vi "FestoCPX.Valve(1out1in).vi"(4 "negate input (F)":bool, 6 "Timeout [ms] (5000)":u32=5000, 8 "error in (no error)":errorcluster, 9 "Position":T3, 10 "Output":T1, 11 "Input":T2) -> (0 "error out":errorcluster, 2 "Aborted?":bool, 3 "Timeout?":bool)   [LabVIEW 2016]
uses:
  Station/Station.ValvePosition.ctl
  FestoCPX.DI.Signal.ctl
  FestoCPX.DO.Signal.ctl
  FestoCPX.DO.Data.State.Set.vi
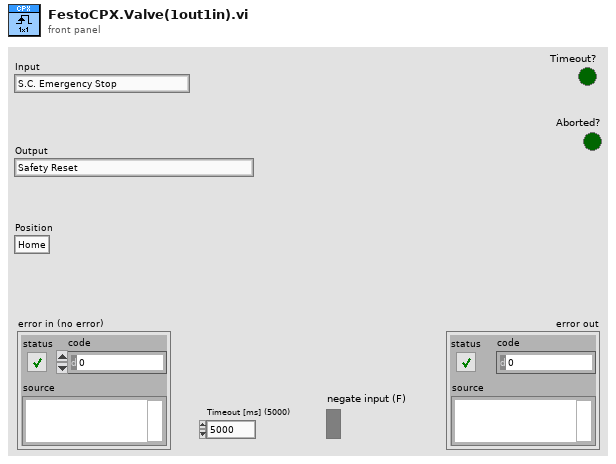
[diagram p1: front panel]
types:
  T1 = typedef "FestoCPX.DO.Signal.ctl" = enum16{"Safety Reset", "Air Main Valve", "Door Lock", "Button LED Start", "Button LED Stop", "Button LED Control", "Traffic LED Red", "Traffic LED Orange", "Traffic LED Green", "Horn", "Laser Interlock", "Laser Trigger", "Laser Fume Extractor", "Product Suction Gripper Slot 1 A", "Product Suction Gripper Slot 1 B", "Product Suction Gripper Slot 2 A", "Product Suction Gripper Slot 2 B", "Product Suction Gripper Slot 3 A", "Product Suction Gripper Slot 3 B", "Product Suction Gripper Slot 4 A", "Product Suction Gripper Slot 4 B", "Product Suction Gripper Final A", "Product Suction Gripper Final B", "Lamp", "Q1 Product Move Work", "Q1 Product Move Home", "Q2 Table Turn Work", "Q2 Table Turn Home", "Q3 Product Lift A", "Q3 Product Lift B", "Q4 Product Arm OK", "Q4 Product Arm NOK", "Q5 Product Arm Work", "Q6 Product BlowOut A", "Q6 Product BlowOut B"}
  T2 = typedef "FestoCPX.DI.Signal.ctl" = enum16{"S.C. Emergency Stop", "S.C. Side Door Close", "S.C. Front Door Close", "S.C. Front Door Secured", "Button Start", "Button Stop", "Button Control", "Product Move Home", "Product Move Work", "Table Position", "Table Lock", "Product Lift A Home", "Product Lift B Home", "Product Arm OK", "Product Arm NOK", "Product Arm Work", "Revolver ID 1", "Revolver ID 2", "Revolver ID 3", "Revolver ID 4", "Revolver ID 5", "Air Pressure Inside", "Air Pressure Inlet", "Product Slot 1 A Present", "Product Slot 1 B Present", "Product Slot 2 A Present", "Product Slot 2 B Present", "Product Slot 3 A Present", "Product Slot 3 B Present", "Product Slot 4 A Present", "Product Slot 4 B Present", "Product Final A Present", "Product Final B Present", "Product Output A Present", "Product Output B Present", "Product Container OK Present", "Product Container NOK Present", "Fork ID 1", "Fork ID 2"}
  T3 = typedef "Station.ValvePosition.ctl" = enum16{"Home", "Work"}
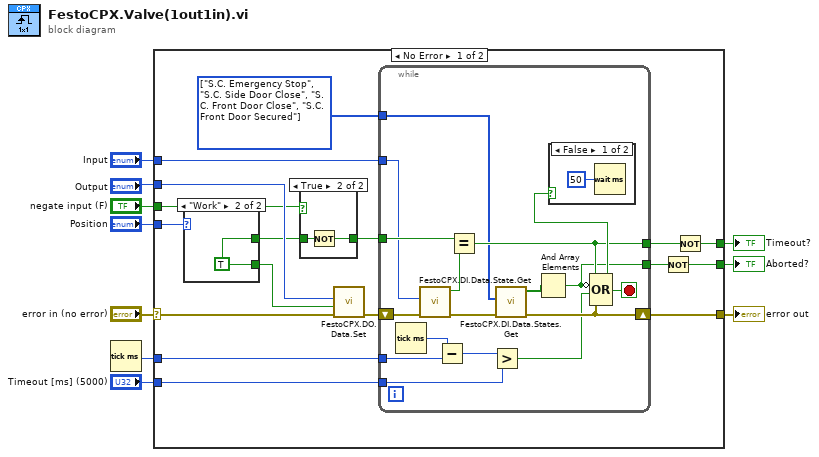
[diagram p0: block diagram]
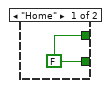
[diagram p3: hidden frame]
diagram:
  n1 = Tick Count (ms)() -> (millisecond timer value=w6:u32)
  n2 = case shown="No Error" "error in (no error)" {
    selector: "error in (no error)" -> [w21 w50]
    tunnel: "Position" -> [w20 _]
    tunnel: [w17 w50] -> w9
    tunnel: [w24 _] -> w8
    tunnel: w6 -> [w27 _]
    tunnel: "Timeout [ms] (5000)" -> [w26 _]
    tunnel: "Input" -> [w25 _]
    tunnel: "Output" -> [w18 _]
    tunnel: [w14 _] -> w2
    tunnel: "negate input (F)" -> [w13 _]
    frame No Error {
      w15 = T2[] [enum."S.C. Emergency Stop", enum."S.C. Side Door Close", enum."S.C. Front Door Close", enum."S.C. Front Door Secured"] items=["S.C. Emergency Stop", "S.C. Side Door Close", "S.C. Front Door Close", "S.C. Front Door Secured", "Button Start", "Button Stop", "Button Control", "Product Move Home", "Product Move Work", "Table Position", "Table Lock", "Product Lift A Home", "Product Lift B Home", "Product Arm OK", "Product Arm NOK", "Product Arm Work", "Revolver ID 1", "Revolver ID 2", "Revolver ID 3", "Revolver ID 4", "Revolver ID 5", "Air Pressure Inside", "Air Pressure Inlet", "Product Slot 1 A Present", "Product Slot 1 B Present", "Product Slot 2 A Present", "Product Slot 2 B Present", "Product Slot 3 A Present", "Product Slot 3 B Present", "Product Slot 4 A Present", "Product Slot 4 B Present", "Product Final A Present", "Product Final B Present", "Product Output A Present", "Product Output B Present", "Product Container OK Present", "Product Container NOK Present", "Fork ID 1", "Fork ID 2"] ("CPX.DI")
      n3 = case shown="\"Work\"" w20 {
        tunnel: [w31 w32] -> w12
        tunnel: [w31 w32] -> w19
        frame "Home" {
          w31 = FALSE
        }
        frame "Work" {
          w32 = TRUE
        }
      }
      n4 = case shown="True" w13 {
        tunnel: w12 -> [w28 w30]
        tunnel: [w28 w29] -> w11
        frame False {
        }
        frame True {
          n5 = Not(x=w30) -> (.not. x?=w29:bool)
        }
      }
      n6 = call-poly "FestoCPX.DO.Data.Set.vi"("error in (no error)"=w21, "State"=w19, "CPX.DO"=w18) -> ("error out"=w23:errorcluster)  [unwired: 8 in]
      n7 = while {
        shift-right: [w37] -> w17
        shift-left: w23 -> [w42]
        tunnel: w25 -> [w40]
        tunnel: [w41] -> w22
        tunnel: w27 -> [w47]
        tunnel: w26 -> [w45]
        tunnel: w11 -> [w44]
        tunnel: [w36] -> w16
        tunnel: w15 -> [w38]
        stop <- w43 stop-if-true
        n8 = Tick Count (ms)() -> (millisecond timer value=w48:u32)
        n9 = call "FestoCPX.DI.Data.State.Get.vi"("error in (no error)"=w42, "CPX.DI"=w40) -> ("error out"=w39:errorcluster, "State"=w33:bool)  [unwired: 5 in, 3 out]
        n10 = Subtract(x=w48, y=w47) -> (x-y=w46:u32)
        n11 = Equal?(x=w44, y=w33) -> (x = y?=w41:bool)
        n12 = Greater?(x=w46, y=w45) -> (0:w35:bool)
        n13 = call "FestoCPX.DI.Data.States.Get.vi"("error in (no error)"=w39, "CPX.DI"=w38) -> ("error out"=w37:errorcluster, "State"=w34:bool[])  [unwired: 5 in, 3 out]
        n14 = And Array Elements(Boolean array=w34) -> (logical AND=w36:bool)
        n15 = Compound Arithmetic op=OR(w41, invert w36, w35, w37) -> (w43:bool)
        n16 = case shown="False" w43 {
          frame False {
            n17 = Wait (ms)(milliseconds to wait=u32 50) -> ()  [unwired: 1 out]
          }
          frame True {
          }
        }
      }
      n18 = Not(x=w16) -> (.not. x?=w14:bool)
      n19 = Not(x=w22) -> (.not. x?=w24:bool)
    }
    frame Error {
    }
  }
  "error out" <- w9
  "Timeout?" <- w8
  "Aborted?" <- w2
